vi "encodeObject.vi"(8 "error in (no error)":errorcluster, 10 "Variant":variant) -> (0 "error out":errorcluster, 2 "Array":u8[](array[numeric]) format="%.0x")   [LabVIEW 2016, in "MsgPack.lvlib"]
uses:
  MsgPack.lvlib
  <vilib>/Utility/error.llb/Error Cluster From Error Code.vi
  <vilib>/ErrorRing/Error Ring.xnode
  <vilib>/Utility/Data Type/NI_Data Type.lvlib
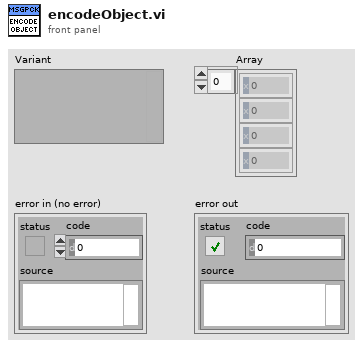
[diagram p1: front panel]
types:
  T1 = typedef "NI_Data Type.lvlib/Data Type.ctl" = enum8{"Invalid Type", "Void", "I8", "I16", "I32", "I64", "U8", "U16", "U32", "U64", "Single Float", "Double Float", "Extended Float", "Single Complex", "Double Complex", "Extended Complex", "Enum U8", "Enum U16", "Enum U32", "Enum U64", "Single Float With Unit", "Double Float With Unit", "Extended Float With Unit", "Single Complex with Unit", "Double Complex with Unit", "Extended Complex with Unit", "Boolean", "String", "Path", "Picture", "Tag", "Array", "Cluster", "Variant", "LV Variant", "Waveform", "Timestamp", "Digital Waveform", "Digital Data", "ExpressData", "Refnum", "External Data", "VI", "Poly VI", "LabVIEW Class Instance", "Fixed Point"}
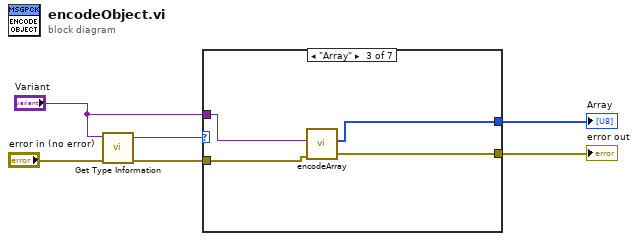
[diagram p0: block diagram]
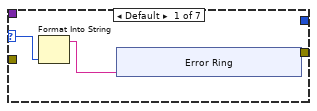
[diagram p2: hidden frame]
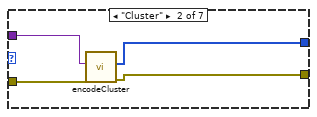
[diagram p3: hidden frame]
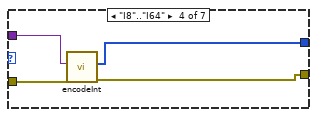
[diagram p4: hidden frame]
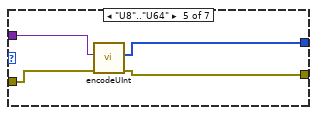
[diagram p5: hidden frame]
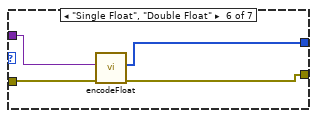
[diagram p6: hidden frame]
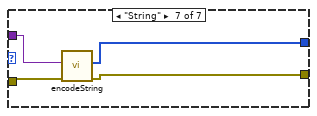
[diagram p7: hidden frame]
diagram:
  n1 = call <vilib>:"Get Type Information.vi"("error in (no error)"="error in (no error)", "Variant"="Variant") -> ("error out"=w4:errorcluster, "Type"=w5:T1)  [unwired: 5 in, 3 out]
  n2 = case shown="\"Array\"" w5 {
    selector: w5 -> [w8 _ _ _ _ _ _]
    tunnel: w4 -> [_ w20 w24 w28 w32 w36 w40]
    tunnel: "Variant" -> [_ w19 w23 w27 w31 w35 w39]
    tunnel: [w9 w18 w21 w25 w30 w33 w37] -> w2
    tunnel: [_ w17 w22 w26 w29 w34 w38] -> w1
    frame Default {
      n3 = Format Into String(w8) -> (resulting string=w7:string)  [unwired: 3 in, 1 out]
      n4 = xnode "Error Ring"("parameter 0"=w7) -> ("error out"=w9:errorcluster)
    }
    frame "Cluster" {
      n5 = call "encodeCluster.vi"("error in (no error)"=w20, "Variant"=w19) -> ("error out"=w18:errorcluster, "Array"=w17:u8[])  [unwired: 8 in]
    }
    frame "Array" {
      n6 = call "encodeArray.vi"("error in (no error)"=w24, "Variant"=w23) -> ("error out"=w21:errorcluster, "Array"=w22:u8[])  [unwired: 8 in]
    }
    frame "I8".."I64" {
      n7 = call "encodeInt.vi"("error in (no error)"=w28, "Variant"=w27) -> ("error out"=w25:errorcluster, "Array"=w26:u8[])  [unwired: 8 in]
    }
    frame "U8".."U64" {
      n8 = call "encodeUInt.vi"("error in (no error)"=w32, "Variant"=w31) -> ("error out"=w30:errorcluster, "Array"=w29:u8[])  [unwired: 8 in]
    }
    frame "Single Float", "Double Float" {
      n9 = call "encodeFloat.vi"("error in (no error)"=w36, "Variant"=w35) -> ("error out"=w33:errorcluster, "Array"=w34:u8[])  [unwired: 8 in]
    }
    frame "String" {
      n10 = call "encodeString.vi"("error in (no error)"=w40, "Variant"=w39) -> ("error out"=w37:errorcluster, "Array"=w38:u8[])  [unwired: 8 in]
    }
  }
  "Array" <- w1
  "error out" <- w2
